vi "Find Regulation Target Crossing.vi"(0 "measurement configuration":T3 {"acq sampling rate" format="%0.2f"; "master clock rate" format="%#_6pHz"; "frame clock rate" format="%#_6pHz"}, 2 "regaultion settings":T14={"enable regulation"=FALSE, "regulation target"=enum."THD+N Ratio", "regulation target value"=0.05, "regulation target value units"=enum."%", "regulation start level"=10.0, "regulation stop level"=70.0, "regulation number of steps"=2}, 5 "error in (no error)":errorcluster, 7 "PCM tasks":T1, 9 "DAQmx task in":refnum<k21>) -> (11 "PCM tasks":T1, 13 "DAQmx task out":refnum<k21>, 14 "measurement configuration out":T3={"digital channel list"="7821\\PCMo 8", "frame clock rate"=48000.0, "number of channels"=2, "channel length"=32, "bit depth"=24, "data justification"=enum."Left Justified", "endianness"=enum."MSB First", "bit clock edge sync"=enum."Falling", "frame sync edge for channel 0"=enum."Falling", "channel 0 offset"=1, "master clock channel list"="7821\\PCMo 0", "master clock rate"=12288000.0, "enable dither"=TRUE, "logic level"=enum."3.3 V", "signal frequency"=1000.0, "output level"=-1.0, "output level units"=enum."dBFS", "output range (pk-pk)"=15.0, "load impedance"=4.0, "signal phase"=0.0, "acq sampling rate"=51200.0, "min measurement cycles"=20, "min measurement time (s)"=0.1, "min settling cycles"=0, "min settling time (s)"=0.0, "acq channel"="", "band start"=20.0, "band stop"=20000.0, "weighting filter"=enum."A-weighting", "highpass filter"=enum."DC", "lowpass filter"=enum."No filter", "SNR units"=enum."dB", "THD+N units"=enum."dB", "THD units"=enum."dB", "gain units"=enum."dB"} {"acq sampling rate" format="%0.2f"; "master clock rate" format="%#_6pHz"; "frame clock rate" format="%#_6pHz"}, 16 "crossing found?":bool, 17 "search results":cluster{"level":dbl, "value":dbl}[](array[cluster]), 19 "error out":errorcluster)   [LabVIEW 2021]
uses:
  controls/single tone measurement settings (HW).ctl
  controls/digital audio protocol/data justification.ctl
  controls/digital audio protocol/endianness.ctl
  controls/digital audio protocol/digital edge.ctl
  controls/digital audio protocol/logic level.ctl
  controls/digital output level units.ctl
  controls/weighting filter.ctl
  controls/highpass filter.ctl
  controls/lowpass filter.ctl
  controls/units - snr.ctl
  controls/units - ratio.ctl
  controls/regulation settings.ctl
  controls/regulation target.ctl
  controls/regulation target value units.ctl
  controls/audio controls.lvlib
  <vilib>/PDM Acquisition Toolkit/host/Classes/Tasks/PCM Output/PCM Output Task.lvclass
  <vilib>/PDM Acquisition Toolkit/host/Classes/Tasks/PCM Output/Controls/PCM Output Task DVR.ctl
  controls/digital audio protocol/PCM tasks.ctl
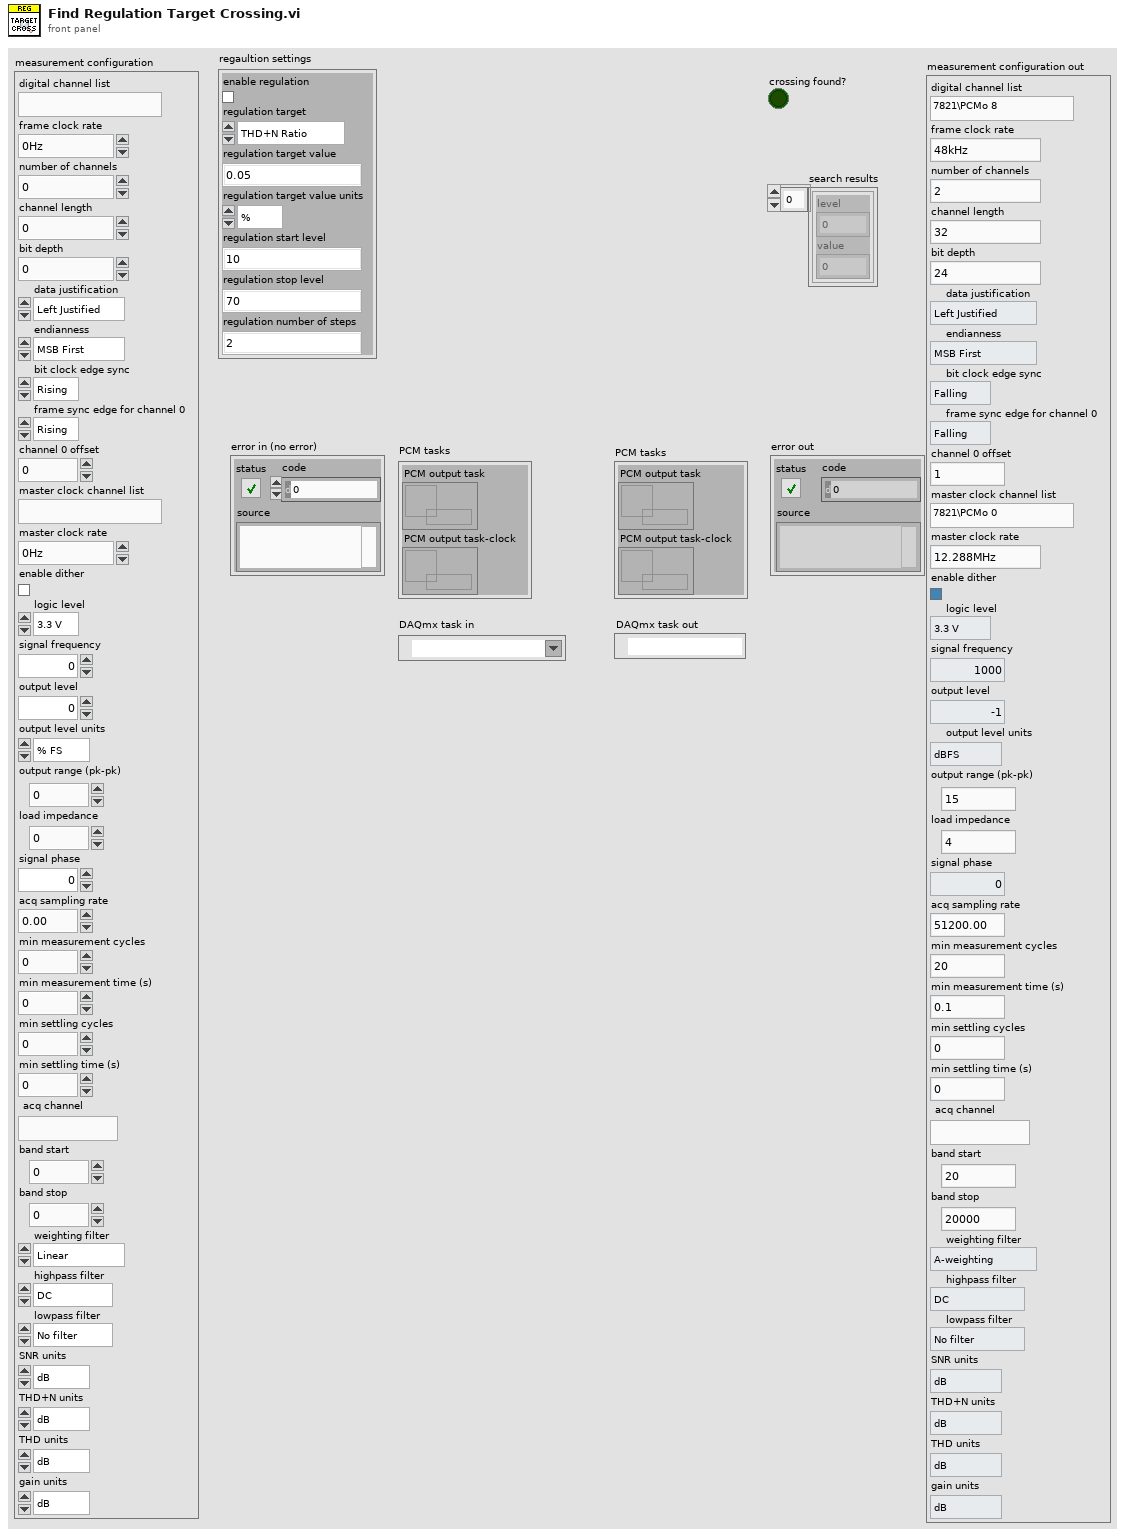
[diagram p1: front panel]
types:
  T1 = typedef "PCM tasks.ctl" = cluster{"PCM output task":T2, "PCM output task-clock":T2}
  T2 = typedef "PDM Acquisition Class Library.lvlib/PCM Output Task.lvclass/PCM Output Task DVR.ctl" = refnum<data-value>
  T3 = typedef "single tone measurement settings (HW).ctl" = cluster{"digital channel list":string, "frame clock rate":dbl, "number of channels":u32, "channel length":u32, "bit depth":u32, "data justification":T4, "endianness":T5, "bit clock edge sync":T6, "frame sync edge for channel 0":T6, "channel 0 offset":u32, "master clock channel list":string, "master clock rate":dbl, "enable dither":bool, "logic level":T7, "signal frequency":dbl, "output level":dbl, "output level units":T8, "output range (pk-pk)":dbl, "load impedance":dbl, "signal phase":dbl, "acq sampling rate":dbl, "min measurement cycles":u32, "min measurement time (s)":dbl, "min settling cycles":u32, "min settling time (s)":dbl, "acq channel":string, "band start":dbl, "band stop":dbl, "weighting filter":T9, "highpass filter":T10, "lowpass filter":T11, "SNR units":T12, "THD+N units":T13, "THD units":T13, "gain units":T13}
  T4 = typedef "data justification.ctl" = enum32{"Left Justified", "Right Justified"}
  T5 = typedef "endianness.ctl" = enum32{"MSB First", "LSB First"}
  T6 = typedef "digital edge.ctl" = enum32{"Rising", "Falling"}
  T7 = typedef "logic level.ctl" = enum32{"3.3 V", "1.8 V", "1.2 V"}
  T8 = typedef "audio controls.lvlib/digital output level units.ctl" = enum32{"% FS", "dBFS", "V"}
  T9 = typedef "weighting filter.ctl" = enum32{"Linear", "A-weighting", "B-weighting", "C-weighting"}
  T10 = typedef "highpass filter.ctl" = enum32{"DC", "AC"}
  T11 = typedef "lowpass filter.ctl" = enum32{"No filter", "AES17 20kHz", "AES17 40kHz"}
  T12 = typedef "audio controls.lvlib/units - snr.ctl" = enum32{"dB", "x/y"}
  T13 = typedef "audio controls.lvlib/units - ratio.ctl" = enum32{"dB", "%", "x/y"}
  T14 = typedef "regulation settings.ctl" = cluster{"enable regulation":bool, "regulation target":T15, "regulation target value":dbl, "regulation target value units":T16, "regulation start level":dbl, "regulation stop level":dbl, "regulation number of steps":u32}
  T15 = typedef "regulation target.ctl" = enum32{"THD+N Ratio", "Output Power"}
  T16 = typedef "regulation target value units.ctl" = enum32{"%", "W"}
  T17 = typedef "audio controls.lvlib/single tone audio measurements.ctl" = cluster{"channel":string, "frequency (Hz)":dbl, "amplitude (Vrms)":dbl, "amplitude (dBFS)":dbl, "phase (deg)":dbl, "SNR":dbl, "THD+N":dbl, "THD":dbl, "dynamic range (dB)":dbl, "gain":dbl, "SFDR (dBc)":dbl}
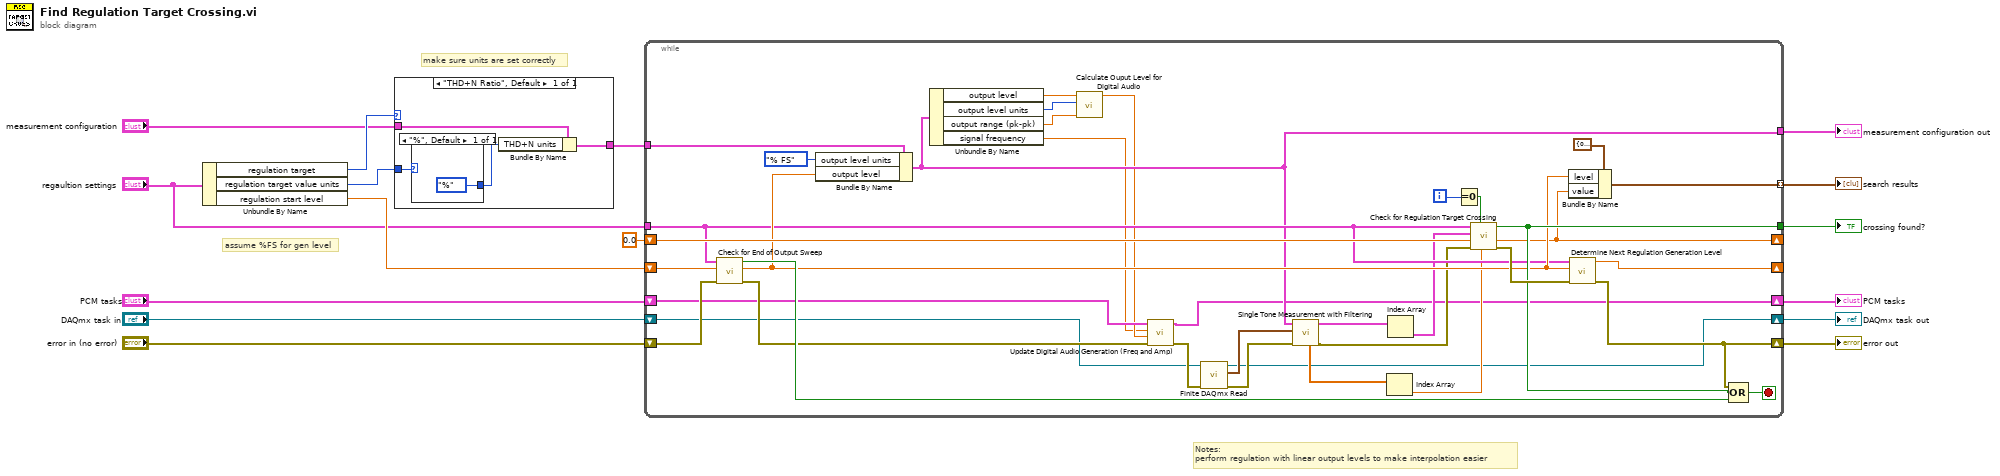
[diagram p0: block diagram]
diagram:
  # "make sure units are set correctly"
  # "assume %FS for gen level"
  # "Notes:\nperform regulation with linear output levels to make interpolation easier"
  n1 = Unbundle By Name("regaultion settings") -> ("regulation target"=w12:T15, "regulation target value units"=w10:T16, "regulation start level"=w14:dbl)
  n2 = case shown="\"THD+N Ratio\", Default" w12 {
    tunnel: [w20] -> w13
    tunnel: "measurement configuration" -> [w18]
    tunnel: w10 -> [w17]
    frame "THD+N Ratio", Default {
      n3 = case shown="\"%\", Default" w17 {
        tunnel: [units_-_ratio."%" ("THD+N units")] -> w19
        frame "%", Default {
        }
      }
      n4 = Bundle By Name(cluster=w18, "THD+N units"=w19) -> (w20:T3)
    }
  }
  n5 = while {
    shift-right: [w50] -> w16
    shift-left: "error in (no error)" -> [w52]
    shift-right: [w54] -> _
    shift-left: w14 -> [w53]
    tunnel: w13 -> [w51]
    shift-right: [w43] -> _
    shift-left: 0.0 ("measured value") -> [w46]
    tunnel: [w47] -> w8
    tunnel: [w42] -> w7 mode=indexing
    tunnel: [w27] -> w5
    tunnel: "regaultion settings" -> [w41]
    shift-right: [w25] -> w2
    shift-left: "PCM tasks" -> [w31]
    shift-right: [w22] -> w1
    shift-left: "DAQmx task in" -> [w30]
    i -> [w57]
    stop <- w48 stop-if-true
    n6 = call "Check for End of Output Sweep.vi"("error in (no error)"=w52, "current generation level"=w53, "regaultion settings"=w41) -> ("error out"=w32:errorcluster, "generation level"=w44:dbl, "sweep done"=w49:bool)  [unwired: 6 in]
    n7 = Bundle By Name(cluster=w51, "output level units"=digital_output_level_units."% FS", "output level"=w44) -> (w27:T3)
    n8 = Unbundle By Name(w27) -> ("output level"=w38:dbl, "output level units"=w37:T8, "output range (pk-pk)"=w36:dbl, "signal frequency"=w23:dbl)
    n9 = call "Calculate Ouput Level for Digital Audio.vi"("output range (pk-pk)"=w36, "digital output level units"=w37, "output level"=w38) -> ("gain"=w24:dbl)  [unwired: 7 in, 1 out]
    n10 = call "Update Digital Audio Generation (Freq and Amp).vi"("error in (no error)"=w32, "gain"=w24, "frequency"=w23, "PCM tasks"=w31) -> ("error out"=w35:errorcluster, "PCM tasks"=w25:T1)  [unwired: 6 in]
    n11 = call "Finite DAQmx Read.vi"("error in (no error)"=w35, "task/channels in"=w30) -> ("error out"=w34:errorcluster, "data"=w33:waveform(dbl)[], "task out"=w22:refnum<k21>)  [unwired: 7 in]
    n12 = call "Single Tone Measurement with Filtering.vi"("error in (no error)"=w34, "waveforms"=w33, "measurement configuration"=w27) -> ("error out"=w26:errorcluster, "results"=w28:T17[], "output power"=w29:dbl[])  [unwired: 4 in, 2 out]
    n13 = Index Array(array=w29) -> (element=w39:dbl)  [unwired: 1 in]
    n14 = Index Array(array=w28) -> (element=w40:T17)  [unwired: 1 in]
    n15 = Equal To 0?(x=w57) -> (x = 0?=w56:bool)
    n16 = call "Check for Regulation Target Crossing.vi"("output power"=w39, "first call?"=w56, "error in (no error)"=w26, "previous measured value"=w46, "results"=w40, "regulation settings"=w41) -> ("error out"=w55:errorcluster, "measured value"=w43:dbl, "crossing found?"=w47:bool)  [unwired: 3 in]
    n17 = Bundle By Name(cluster=cluster{"level":dbl, "value":dbl} {"level"=0.0, "value"=0.0}, "level"=w44, "value"=w43) -> (w42:cluster{"level":dbl, "value":dbl})
    n18 = call "Determine Next Regulation Generation Level.vi"("error in (no error)"=w55, "current generation level"=w44, "regulation settings"=w41) -> ("error out"=w50:errorcluster, "next generation level"=w54:dbl)  [unwired: 7 in]
    n19 = Compound Arithmetic op=OR(w50, w47, w49) -> (w48:bool)
  }
  "error out" <- w16
  "crossing found?" <- w8
  "search results" <- w7
  "measurement configuration out" <- w5
  "PCM tasks" <- w2
  "DAQmx task out" <- w1
